vi "run.vi"(11 "noncancellable wait in":refnum<class "noncancellable wait.lvclass">) -> (2 "result":refnum<class "result.lvclass">, 3 "noncancellable wait out":refnum<class "noncancellable wait.lvclass">)   [LabVIEW 2013, in "noncancellable wait.lvclass"]
uses:
  noncancellable wait.lvclass
  result/result.lvclass
  noncancellable wait.lvclass/noncancellable wait.ctl
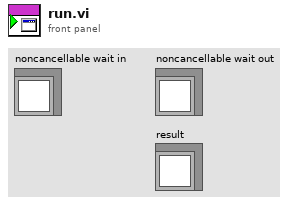
[diagram p1: front panel]
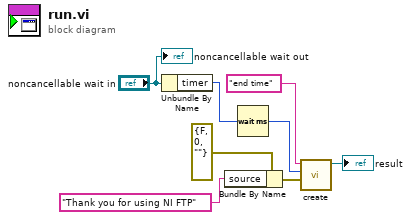
[diagram p0: block diagram]
diagram:
  n1 = Unbundle By Name("noncancellable wait in") -> ("timer"=w3:i32)
  n2 = Bundle By Name(cluster=errorcluster {"status"=FALSE, "code"=0, "source"=""} ("error constant"), "source"="Thank you for using NI FTP") -> (w7:errorcluster)
  n3 = Wait (ms)(milliseconds to wait=w3) -> (millisecond timer value=w5:u32)
  n4 = call "create.vi"("error"=w7, "data"=w5, "data ID"="end time") -> ("result out"=→"result":refnum<class "result.lvclass">)  [unwired: 8 in]
  "noncancellable wait out" <- "noncancellable wait in"
